vi "Create 1 Hidden Layer.vi"(0 "1st Hidden Layer Neurons":u32, 1 "Output Layer Linear":bool, 2 "Add Bias Inputs":bool=TRUE, 11 "Error In":errorcluster, 12 "# Inputs":u32, 13 "Output Neurons/Outputs":u32) -> (4 "Neural Network Out":T1={"Weigths"=[], "Last Layer Linear"=TRUE, "Add Bias Inputs"=TRUE, "# Inputs"=0, "# Output Neurons/Outputs"=0, "Inputs Scaling"={"X Scaling Vector"=[], "Y Scaling Vector"=[]}, "Outputs Scaling"={"X Scaling Vector"=[], "Y Scaling Vector"=[]}}, 15 "Error Out":errorcluster)   [LabVIEW 2013, in "Super Simple Neural Network.lvlib"]
doc: "Experiment and theory shows that one hidden layer is enough to solve most problems presented to neural networks. If you see that one hidden layer is not enough you have an option to choose two hidden layers initializer. \n\nThis VI creates a neural network with 1 hidden layer. This means that the network has 3 layers: input, hidden and output. Networks implement scaling of input and output values to the range of 0.2 to 0.8. This makes the unipolar sigmoidal activation function of the neurons most effective.\n\n<b> Add Bias Inputs</b> - this setting adds bias inputs of 1 to all neurons of all layers. This greatly imroves the performance of the teaching algorithm.\n\n<b>1st Hidden Layer</b> - experiments show that number of hidden neurons close to sqrt(2) * n where n is the number of inputs is in most cases optimal for the size of the network.\n\n<b> Output Layer Linear</b> - If the output values that you want to get from the network are not bound by max and min values you should set the output layer to linear. This setting allows the network to output effectivly beyond the range of values that you teach it with."
uses:
  Super Simple Neural Network.lvlib
  Types/Neural Network.ctl
  Types/2D Array.ctl
  Types/Scaling Info.ctl
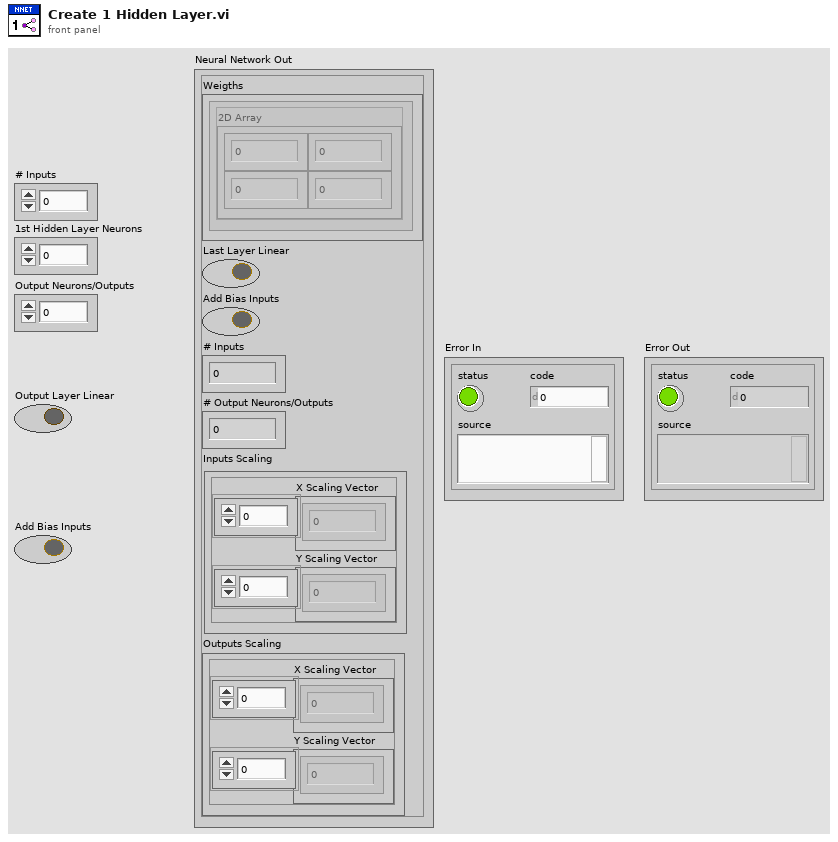
[diagram p1: front panel]
types:
  T1 = typedef "Super Simple Neural Network.lvlib/Neural Network.ctl" = cluster{"Weigths":T2[], "Last Layer Linear":bool, "Add Bias Inputs":bool, "# Inputs":u32, "# Output Neurons/Outputs":u32, "Inputs Scaling":T3, "Outputs Scaling":T3}
  T2 = typedef "Super Simple Neural Network.lvlib/2D Array.ctl" = cluster{"2D Array":dbl[][]}
  T3 = typedef "Super Simple Neural Network.lvlib/Scaling Info.ctl" = cluster{"X Scaling Vector":dbl[], "Y Scaling Vector":dbl[]}
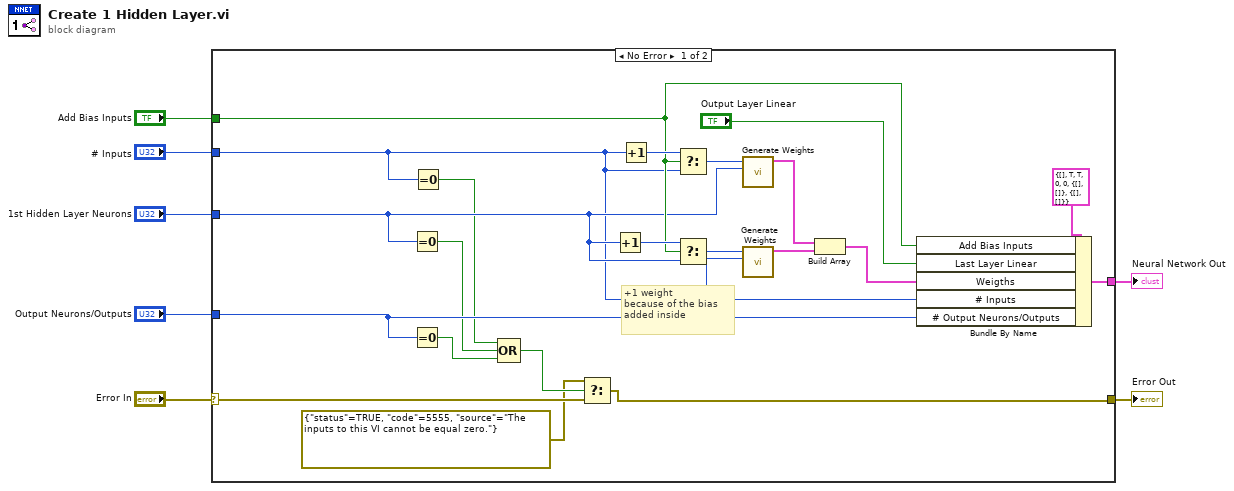
[diagram p0: block diagram]
diagram:
  n1 = case shown="No Error" "Error In" {
    selector: "Error In" -> [w10 w29]
    tunnel: [w27 _] -> w7
    tunnel: "Output Neurons/Outputs" -> [w17 _]
    tunnel: "# Inputs" -> [w15 _]
    tunnel: "Add Bias Inputs" -> [w21 _]
    tunnel: "1st Hidden Layer Neurons" -> [w16 _]
    tunnel: [w8 w29] -> w1
    frame No Error {
      # "+1 weight\nbecause of the bias\nadded inside"
      n2 = Equal To 0?(x=w16) -> (x = 0?=w13:bool)
      n3 = Equal To 0?(x=w17) -> (x = 0?=w14:bool)
      n4 = Equal To 0?(x=w15) -> (x = 0?=w12:bool)
      n5 = Compound Arithmetic op=OR(w12, w13, w14) -> (w11:bool)
      n6 = Select(t=errorcluster {"status"=TRUE, "code"=5555, "source"="The inputs to this VI cannot be equal zero."}, s=w11, f=w10) -> (s? t:f=w8:errorcluster)
      n7 = Increment(x=w16) -> (x+1=w24:u32)
      n8 = Increment(x=w15) -> (x+1=w22:u32)
      n9 = Select(t=w22, s=w21, f=w15) -> (s? t:f=w20:u32)
      n10 = Select(t=w24, s=w21, f=w16) -> (s? t:f=w23:u32)
      n11 = call "Generate Weights.vi"("Neurons"=w16, "Inputs"=w20) -> ("Layer Weights"=w19:T2)  [unwired: 9 in]
      n12 = call "Generate Weights.vi"("Neurons"=w17, "Inputs"=w23) -> ("Layer Weights"=w28:T2)  [unwired: 9 in]
      n13 = Build Array(w19, w28) -> (w18:T2[])
      n14 = Bundle By Name(cluster=T1 {"Weigths"=[], "Last Layer Linear"=TRUE, "Add Bias Inputs"=TRUE, "# Inputs"=0, "# Output Neurons/Outputs"=0, "Inputs Scaling"={"X Scaling Vector"=[], "Y Scaling Vector"=[]}, "Outputs Scaling"={"X Scaling Vector"=[], "Y Scaling Vector"=[]}} ("Neural Network"), "Add Bias Inputs"=w21, "Last Layer Linear"="Output Layer Linear", "Weigths"=w18, "# Inputs"=w15, "# Output Neurons/Outputs"=w17) -> (w27:T1)
    }
    frame Error {
    }
  }
  "Neural Network Out" <- w7
  "Error Out" <- w1
